vi "image size converter.vi"() -> ()   [LabVIEW 2010]
panel:
  out "return code":i32
  out "concatenated string":string
  out "error out 2":errorcluster
  out "standard error 2":string
  out "standard output 2":string
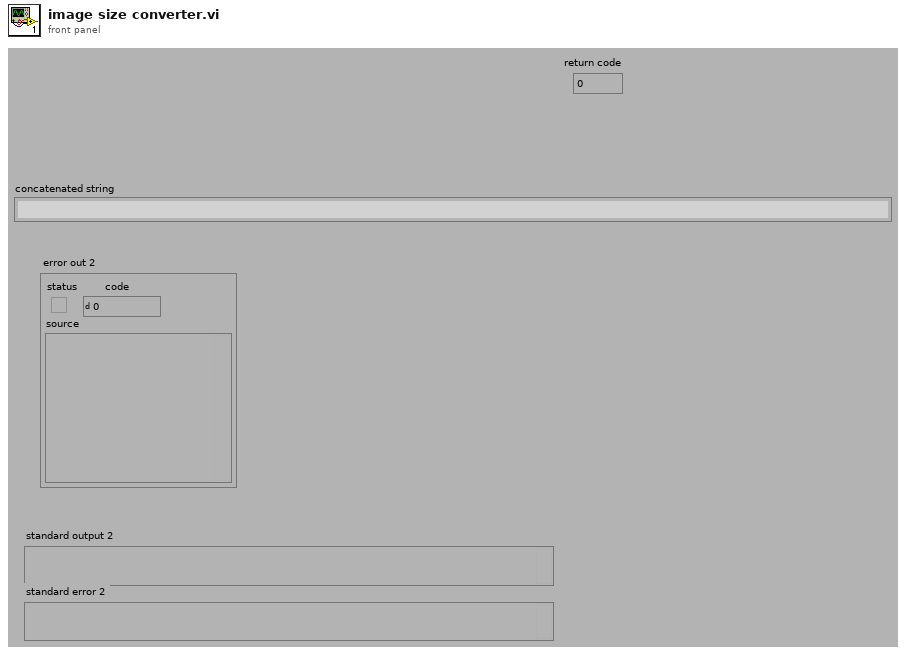
[diagram p1: front panel]
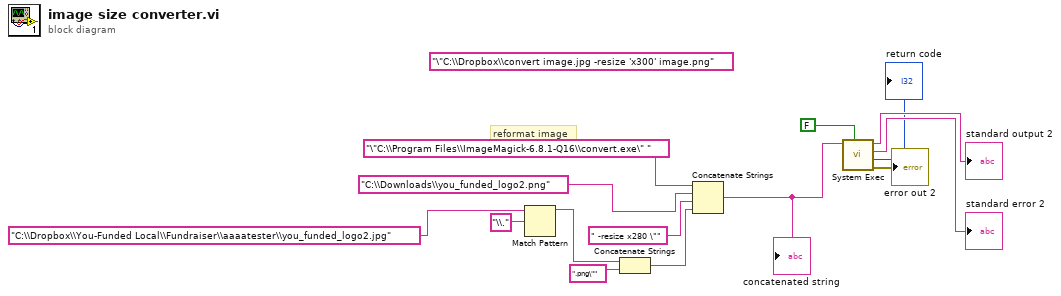
[diagram p0: block diagram]
diagram:
  (unwired) "\"C:\\Dropbox\\convert image.jpg -resize 'x300' image.png" ("command line")
  # "reformat image"
  n1 = Match Pattern(string="C:\\Dropbox\\You-Funded Local\\Fundraiser\\aaaatester\\you_funded_logo2.jpg", regular expression="\\.") -> (before substring=w9:string)  [unwired: 1 in, 3 out]
  n2 = Concatenate Strings(w9, ".png\"" ("string")) -> (w5:string)
  n3 = Concatenate Strings("\"C:\\Program Files\\ImageMagick-6.8.1-Q16\\convert.exe\" " ("string"), "C:\\Downloads\\you_funded_logo2.png" ("string"), " -resize x280 \"" ("string"), w5) -> (w1:string)
  "concatenated string" <- w1
  n4 = call <vilib>:"System Exec.vi"("wait until completion? (T)"=FALSE, "command line"=w1) -> ("error out"=→"error out 2":errorcluster, "return code"=→"return code":i32, "standard error"=→"standard error 2":string, "standard output"=→"standard output 2":string)  [unwired: 6 in]
